vi "Vision Processing.vi"(4 "error in (no error)":errorcluster, 7 "Front Image Size":T1=enum."320x240") -> ()   [LabVIEW 2016]
doc: "This VI runs in parallel to other tasks. It gets images from the camera, processes them for color or shape and use that information to affect robot behavior."
uses:
  <vilib>/Rock Robotics/WPI/Camera/WPI_CameraImageSize.ctl
  <vilib>/Rock Robotics/WPI/Camera/WPI_CameraWhite Balance Values.ctl
  <vilib>/Rock Robotics/WPI/Camera/WPI_CameraExposure Values.ctl
  <vilib>/Rock Robotics/WPI/Camera/WPI_CameraFrameRate.ctl
  Robot Global Data.vi
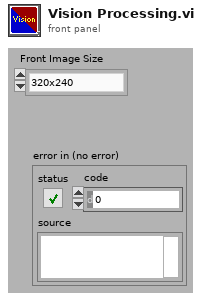
[diagram p1: front panel]
types:
  T1 = typedef "WPI_CameraImageSize.ctl" = enum16{"640x480", "320x240", "160x120", "Custom"}
  T2 = typedef "WPI_CameraFrameRate.ctl" = u32
  T3 = typedef "WPI_CameraExposure Values.ctl" = enum16{"Auto", "Flicker-free 50 Hz", "Flicker-free 60 Hz", "Hold current", "Custom"}
  T4 = typedef "WPI_CameraWhite Balance Values.ctl" = enum16{"Auto", "Fixed indoor", "Fixed outdoor 1", "Fixed outdoor 2", "Fixed fluorescent 1", "Fixed fluorescent 2", "Hold current", "Custom"}
  T5 = typedef "WPI_CameraDevRef.ctl" = cluster{"Camera Address":string, "CameraStatus":errorcluster}
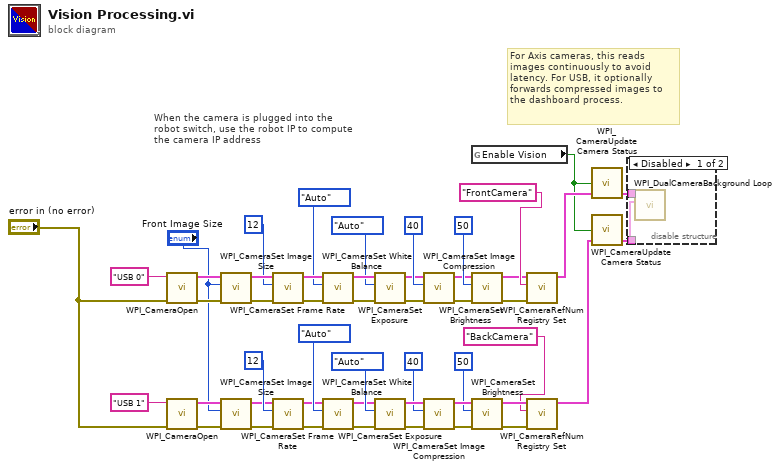
[diagram p0: block diagram]
diagram:
  # "When the camera is plugged into the\nrobot switch, use the robot IP to compute\nthe camera IP address"
  # "For Axis cameras, this reads\nimages continuously to avoid\nlatency. For USB, it optionally\nforwards compressed images to\nthe dashboard process."
  n1 = call <vilib>:"WPI_CameraOpen.vi"("error in (no error)"="error in (no error)", "Camera Address"="USB 0" ("format string")) -> ("error out"=w40:errorcluster, "CameraDevRef"=w41:T5)  [unwired: 8 out]
  n2 = call <vilib>:"WPI_CameraOpen.vi"("error in (no error)"="error in (no error)", "Camera Address"="USB 1" ("format string")) -> ("error out"=w19:errorcluster, "CameraDevRef"=w18:T5)  [unwired: 8 out]
  n3 = call <vilib>:"WPI_CameraSet Image Size.vi"("error in (no error)"=w40, "Image Size"="Front Image Size", "CameraDevRef"=w41) -> ("error out"=w39:errorcluster, "CameraDevRef Out"=w42:T5)  [unwired: 1 in, 6 out]
  n4 = call <vilib>:"WPI_CameraSet Image Size.vi"("error in (no error)"=w19, "Image Size"="Front Image Size", "CameraDevRef"=w18) -> ("error out"=w20:errorcluster, "CameraDevRef Out"=w17:T5)  [unwired: 1 in, 6 out]
  n5 = call <vilib>:"WPI_CameraSet Frame Rate.vi"("error in (no error)"=w39, "Frame Rate (fps)"=T2 12, "CameraDevRef"=w42) -> ("error out"=w38:errorcluster, "CameraDevRef Out"=w44:T5)  [unwired: 7 out]
  n6 = call <vilib>:"WPI_CameraSet Frame Rate.vi"("error in (no error)"=w20, "Frame Rate (fps)"=T2 12, "CameraDevRef"=w17) -> ("error out"=w21:errorcluster, "CameraDevRef Out"=w15:T5)  [unwired: 7 out]
  n7 = call <vilib>:"WPI_CameraSet White Balance.vi"("error in (no error)"=w38, "White Balance"=WPI_CameraWhite_Balance_Values."Auto", "CameraDevRef"=w44) -> ("error out"=w37:errorcluster, "CameraDevRef Out"=w43:T5)  [unwired: 1 in, 6 out]
  n8 = call <vilib>:"WPI_CameraSet White Balance.vi"("error in (no error)"=w21, "White Balance"=WPI_CameraWhite_Balance_Values."Auto", "CameraDevRef"=w15) -> ("error out"=w22:errorcluster, "CameraDevRef Out"=w16:T5)  [unwired: 1 in, 6 out]
  n9 = call <vilib>:"WPI_CameraSet Exposure.vi"("error in (no error)"=w37, "Exposure"=WPI_CameraExposure_Values."Auto", "CameraDevRef"=w43) -> ("error out"=w36:errorcluster, "CameraDevRef Out"=w46:T5)  [unwired: 1 in, 6 out]
  n10 = call <vilib>:"WPI_CameraSet Exposure.vi"("error in (no error)"=w22, "Exposure"=WPI_CameraExposure_Values."Auto", "CameraDevRef"=w16) -> ("error out"=w23:errorcluster, "CameraDevRef Out"=w13:T5)  [unwired: 1 in, 6 out]
  n11 = call <vilib>:"WPI_CameraSet Image Compression.vi"("error in (no error)"=w36, "Compression"=40, "CameraDevRef"=w46) -> ("error out"=w35:errorcluster, "CameraDevRef Out"=w45:T5)  [unwired: 7 out]
  n12 = call <vilib>:"WPI_CameraSet Image Compression.vi"("error in (no error)"=w23, "Compression"=40, "CameraDevRef"=w13) -> ("error out"=w24:errorcluster, "CameraDevRef Out"=w14:T5)  [unwired: 7 out]
  n13 = global read "Robot Global Data.vi" "Enable Vision"() -> (w3:bool)
  n14 = call <vilib>:"WPI_CameraSet Brightness.vi"("error in (no error)"=w35, "Brightness"=50, "CameraDevRef"=w45) -> ("error out"=w33:errorcluster, "CameraDevRef Out"=w34:T5)  [unwired: 7 out]
  n15 = call <vilib>:"WPI_CameraSet Brightness.vi"("error in (no error)"=w24, "Brightness"=50, "CameraDevRef"=w14) -> ("error out"=w26:errorcluster, "CameraDevRef Out"=w25:T5)  [unwired: 7 out]
  n16 = call <vilib>:"WPI_CameraRefNum Registry Set.vi"("error in (no error)"=w33, "refnum name"="FrontCamera", "CameraDevRef"=w34) -> ("CameraDevRef"=w7:T5)  [unwired: 1 in, 7 out]
  n17 = call <vilib>:"WPI_CameraRefNum Registry Set.vi"("error in (no error)"=w26, "refnum name"="BackCamera", "CameraDevRef"=w25) -> ("CameraDevRef"=w5:T5)  [unwired: 1 in, 7 out]
  n18 = call <vilib>:"WPI_CameraUpdate Camera Status.vi"("CameraDevRef In"=w7, "Enable Vision"=w3) -> ("CameraDevRef Out"=w6:T5)  [unwired: 3 in]
  n19 = call <vilib>:"WPI_CameraUpdate Camera Status.vi"("CameraDevRef In"=w5, "Enable Vision"=w3) -> ("CameraDevRef Out"=w4:T5)  [unwired: 3 in]
  n20 = disable-structure shown="Disabled" {
    disable-tunnel: w6 -> [w51 _]
    disable-tunnel: w4 -> [w50 _]
    frame Disabled {
      n21 = call "WPI_DualCameraBackground Loop.vi"("BackCameraDevRef"=w50, "FrontCameraDevRef"=w51) -> ()  [unwired: 10 in]
    }
    frame Enabled {
    }
  }
